vi "FGV-BroadcastRegistry backup.vi"() -> ()   [LabVIEW 2014]
panel:
  in  "Operation":T1(ring)
  in  "ActingMsg In":string="STATUS"
  out "ActingMsg out":string="STATUS"
  in  "Message":string="STATUS"
  in  "Dest":string="M"
  in  "Source":string="A"
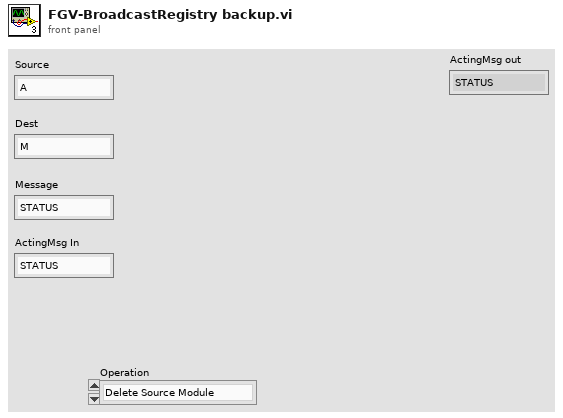
[diagram p1: front panel]
types:
  T1 = enum16{"Delete Source Module", "Delete Dest Module", "Register", "Unregister", "Check"}
  T2 = cluster{"Source":string[], "Dest":string[], "BroadcastMsg":string[], "RegistryTable":string[][][]}
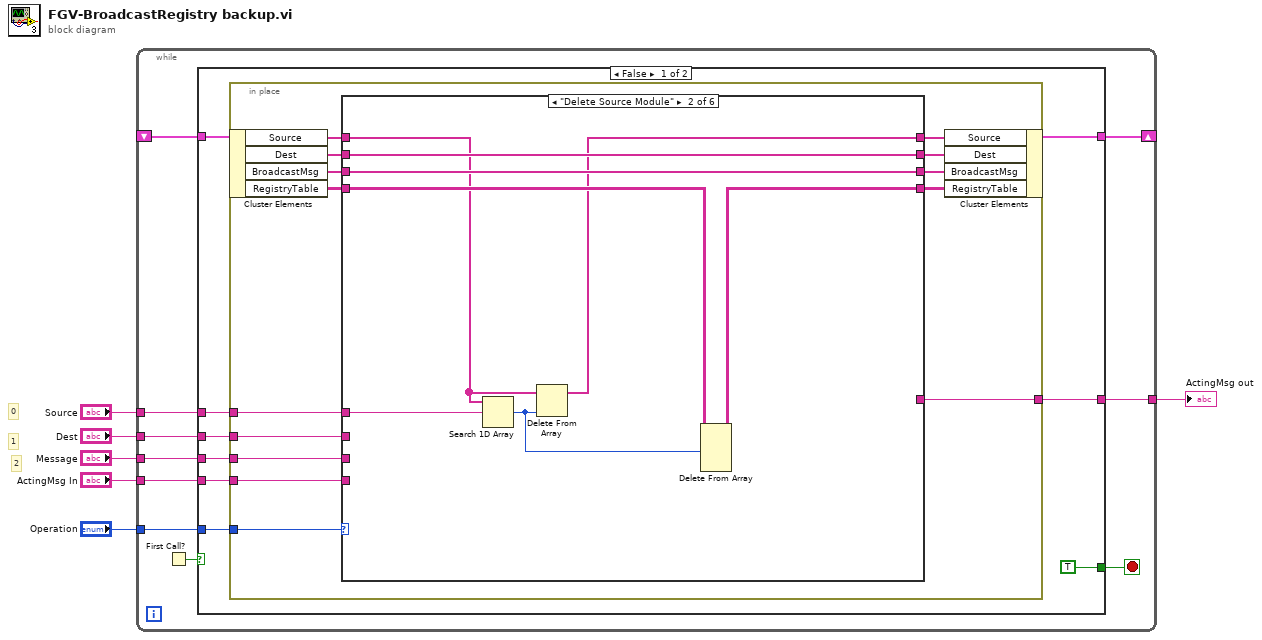
[diagram p0: block diagram]
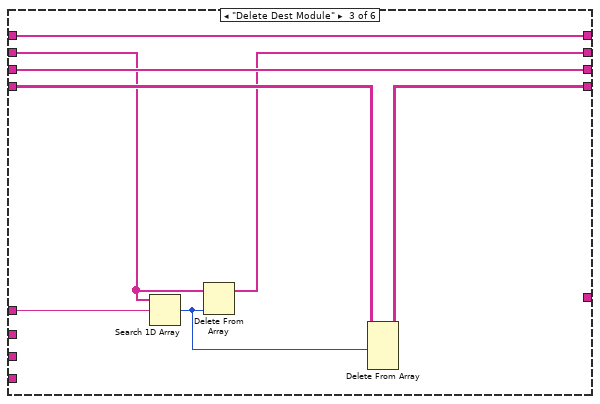
[diagram p3: hidden frame]
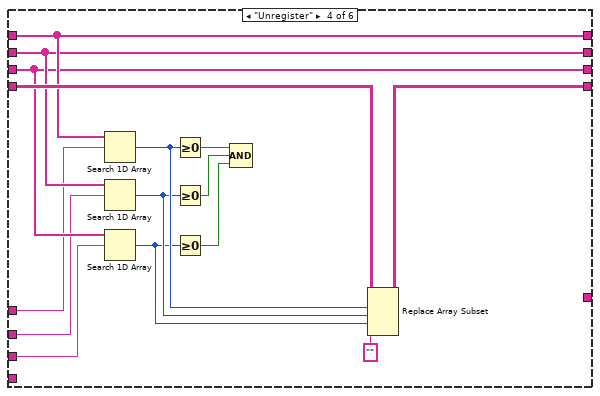
[diagram p4: hidden frame]
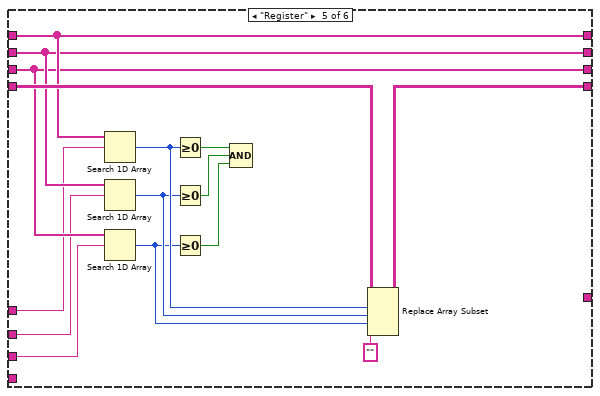
[diagram p5: hidden frame]
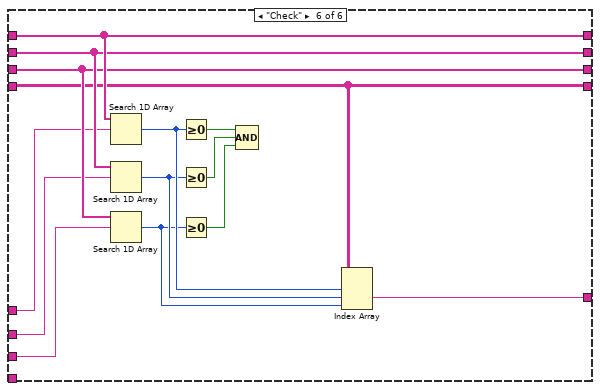
[diagram p6: hidden frame]
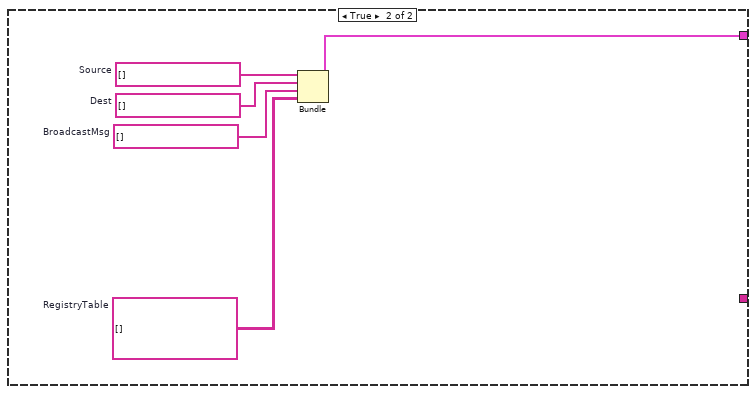
[diagram p7: hidden frame]
diagram:
  # "2"
  # "0"
  # "1"
  n1 = while {
    shift-right: [w14] -> _
    shift-left: _ -> [w13]
    tunnel: "Operation" -> [w12]
    tunnel: "Dest" -> [w11]
    tunnel: "Source" -> [w10]
    tunnel: "Message" -> [w9]
    tunnel: "ActingMsg In" -> [w8]
    tunnel: [w7] -> w1
    stop <- w15 stop-if-true
    n2 = First Call?() -> (First Call?: T/F=w16:bool)
    n3 = case shown="False" w16 {
      tunnel: [TRUE _] -> w15
      tunnel: [w23 w104] -> w14
      tunnel: w13 -> [w24 _]
      tunnel: w12 -> [w22 _]
      tunnel: w11 -> [w21 _]
      tunnel: w10 -> [w20 _]
      tunnel: w9 -> [w19 _]
      tunnel: w8 -> [w18 _]
      tunnel: [w17 _] -> w7
      frame False {
        n4 = in-place {
          in-place-border: w22 -> [w39]
          in-place-border: w21 -> [w30]
          in-place-border: w20 -> [w29]
          in-place-border: w19 -> [w28]
          in-place-border: w18 -> [w27]
          in-place-border: [w26] -> w17
          n5 = in-place-cluster #1(w24) -> ("Source"=w35:string[], "Dest"=w37:string[], "BroadcastMsg"=w33:string[], "RegistryTable"=w31:string[][][])
          n6 = case shown="\"Delete Source Module\"" w39 {
            tunnel: [w42 w46 w52 w68 w83 w102] -> w38
            tunnel: w37 -> [w42 w46 w53 w68 w83 w102]
            tunnel: [w43 w44 w54 w69 w84 w103] -> w36
            tunnel: w35 -> [w43 w45 w54 w69 w84 w103]
            tunnel: [w41 w51 w59 w67 w82 w101] -> w34
            tunnel: w33 -> [w41 w51 w59 w67 w82 w101]
            tunnel: [w40 w49 w57 w73 w88 w94] -> w32
            tunnel: w31 -> [w40 w50 w58 w74 w89 w94]
            tunnel: w30 -> [_ _ _ w65 w80 w99]
            tunnel: w29 -> [_ w48 w56 w66 w81 w100]
            tunnel: w28 -> [_ _ _ w64 w79 w98]
            tunnel: w27 -> [_ _ _ _ _ _]
            tunnel: [_ _ _ _ _ w90] -> w26
            frame Default {
            }
            frame "Delete Source Module" {
              n7 = Search 1D Array(1D array=w45, element=w48) -> (index of element=w47:i32)  [unwired: 1 in]
              n8 = Delete From Array(array=w45, index=w47) -> (array with subset deleted=w44:string[])  [unwired: 1 in, 1 out]
              n9 = Delete From Array(array=w50, index (dim 0)=w47) -> (array with subset deleted=w49:string[][][])  [unwired: 3 in, 1 out]
            }
            frame "Delete Dest Module" {
              n10 = Search 1D Array(1D array=w53, element=w56) -> (index of element=w55:i32)  [unwired: 1 in]
              n11 = Delete From Array(array=w53, index=w55) -> (array with subset deleted=w52:string[])  [unwired: 1 in, 1 out]
              n12 = Delete From Array(array=w58, index (dim 0)=w55) -> (array with subset deleted=w57:string[][][])  [unwired: 3 in, 1 out]
            }
            frame "Unregister" {
              n13 = Search 1D Array(1D array=w69, element=w66) -> (index of element=w63:i32)  [unwired: 1 in]
              n14 = Search 1D Array(1D array=w68, element=w65) -> (index of element=w62:i32)  [unwired: 1 in]
              n15 = Search 1D Array(1D array=w67, element=w64) -> (index of element=w61:i32)  [unwired: 1 in]
              n16 = Greater Or Equal To 0?(x=w63) -> (x >= 0?=w72:bool)
              n17 = Greater Or Equal To 0?(x=w62) -> (x >= 0?=w71:bool)
              n18 = Greater Or Equal To 0?(x=w61) -> (x >= 0?=w70:bool)
              n19 = Compound Arithmetic op=AND(w72, w71, w70) -> ()  [unwired: 1 out]
              n20 = Replace Array Subset(array=w74, new element="" ("new element/subarray"), index (dim 0)=w63, index (dim 1)=w62, index (dim 2)=w61) -> (w73:string[][][])
            }
            frame "Register" {
              n21 = Search 1D Array(1D array=w84, element=w81) -> (index of element=w78:i32)  [unwired: 1 in]
              n22 = Search 1D Array(1D array=w83, element=w80) -> (index of element=w77:i32)  [unwired: 1 in]
              n23 = Search 1D Array(1D array=w82, element=w79) -> (index of element=w76:i32)  [unwired: 1 in]
              n24 = Greater Or Equal To 0?(x=w78) -> (x >= 0?=w87:bool)
              n25 = Greater Or Equal To 0?(x=w77) -> (x >= 0?=w86:bool)
              n26 = Greater Or Equal To 0?(x=w76) -> (x >= 0?=w85:bool)
              n27 = Compound Arithmetic op=AND(w87, w86, w85) -> ()  [unwired: 1 out]
              n28 = Replace Array Subset(array=w89, new element="" ("new element/subarray"), index (dim 0)=w78, index (dim 1)=w77, index (dim 2)=w76) -> (w88:string[][][])
            }
            frame "Check" {
              n29 = Search 1D Array(1D array=w103, element=w100) -> (index of element=w93:i32)  [unwired: 1 in]
              n30 = Search 1D Array(1D array=w102, element=w99) -> (index of element=w92:i32)  [unwired: 1 in]
              n31 = Search 1D Array(1D array=w101, element=w98) -> (index of element=w91:i32)  [unwired: 1 in]
              n32 = Greater Or Equal To 0?(x=w93) -> (x >= 0?=w97:bool)
              n33 = Greater Or Equal To 0?(x=w92) -> (x >= 0?=w96:bool)
              n34 = Greater Or Equal To 0?(x=w91) -> (x >= 0?=w95:bool)
              n35 = Compound Arithmetic op=AND(w97, w96, w95) -> ()  [unwired: 1 out]
              n36 = Index Array(array=w94, index (dim 0)=w93, index (dim 1)=w92, index (dim 2)=w91) -> (element=w90:string)
            }
          }
          n37 = in-place-cluster #1("Source"=w36, "Dest"=w38, "BroadcastMsg"=w34, "RegistryTable"=w32) -> (w23:T2)
        }
      }
      frame True {
        w105 = string[][][] []  # RegistryTable
        w106 = string[] []  # BroadcastMsg
        w107 = string[] []  # Dest
        w108 = string[] []  # Source
        n38 = Bundle("Source"=w108, "Dest"=w107, "BroadcastMsg"=w106, "RegistryTable"=w105) -> (w104:T2)  [unwired: 1 in]
      }
    }
  }
  "ActingMsg out" <- w1
